vi "Test DAQ Synchronize.vi"() -> ()   [LabVIEW 2019, in "Instrument.Lockin.lvlib" / "Instrument.DAQ.lvclass"]
uses:
  Instrument.DAQ.lvclass
  Typedefs/DAQ.Config.AI--Cluster.ctl
  Typedefs/DAQ.Config.AI.Coupling--enum.ctl
  Typedefs/DAQ.Config.AI.Range--enum.ctl
  Typedefs/DAQ.Type--enum.ctl
  Typedefs/DAQ.Config.AO--Cluster.ctl
  Typedefs/DAQ.Config.AO.Range--enum.ctl
  Typedefs/DAQ.Sampling.Sample Mode--Ring.ctl
  Typedefs/DAQ.Sampling.Sampling--Cluster.ctl
  Instrument.DAQ.lvclass/Instrument.DAQ.ctl
  <vilib>/DAQmx/write.llb/DAQmx Write (Analog 1D Wfm NChan NSamp).vi
  <vilib>/DAQmx/read.llb/DAQmx Read (Analog 1D Wfm NChan NSamp).vi
  <vilib>/DAQmx/miscellaneous.llb/DAQmx Fill In Error Info.vi
  <vilib>/measure/NI_MABase.lvlib
  <resource>/objmgr/daqmx.rc
panel:
  out "Waveform Graph":dbl[][](graph)
  in  "stop":bool
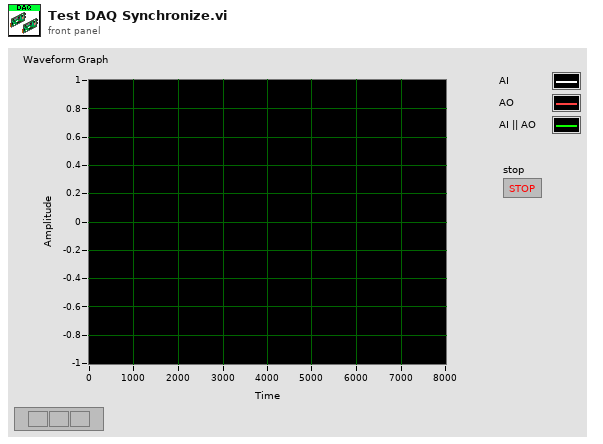
[diagram p1: front panel]
types:
  T1 = typedef "Instrument.Lockin.lvlib/Instrument.DAQ.lvclass/DAQ.Sampling.Sampling--Cluster.ctl" = cluster{"Fs":dbl, "#s":i32}
  T2 = typedef "Instrument.Lockin.lvlib/Instrument.DAQ.lvclass/DAQ.Sampling.Sample Mode--Ring.ctl" = i32
  T3 = typedef "Instrument.Lockin.lvlib/Instrument.DAQ.lvclass/DAQ.Config.AO--Cluster.ctl" = cluster{"Channels":tag, "Range":T4, "output terminal configuration":i32, "Type":T5}
  T4 = typedef "Instrument.Lockin.lvlib/Instrument.DAQ.lvclass/DAQ.Config.AO.Range--enum.ctl" = enum16{"±0.1", "±1.0", "±10.0"}
  T5 = typedef "Instrument.Lockin.lvlib/Instrument.DAQ.lvclass/DAQ.Type--enum.ctl" = enum16{"None", "USB-4431", "PXI-446x"}
  T6 = typedef "Instrument.Lockin.lvlib/Instrument.DAQ.lvclass/DAQ.Config.AI--Cluster.ctl" = cluster{"Channels":tag, "Coupling":T7, "Range":T8, "input terminal configuration":i32, "Type":T5}
  T7 = typedef "Instrument.Lockin.lvlib/Instrument.DAQ.lvclass/DAQ.Config.AI.Coupling--enum.ctl" = u16
  T8 = typedef "Instrument.Lockin.lvlib/Instrument.DAQ.lvclass/DAQ.Config.AI.Range--enum.ctl" = enum16{"±0.316", "±1.00", "±3.16", "±10.0", "±31.6", "±42.4"}
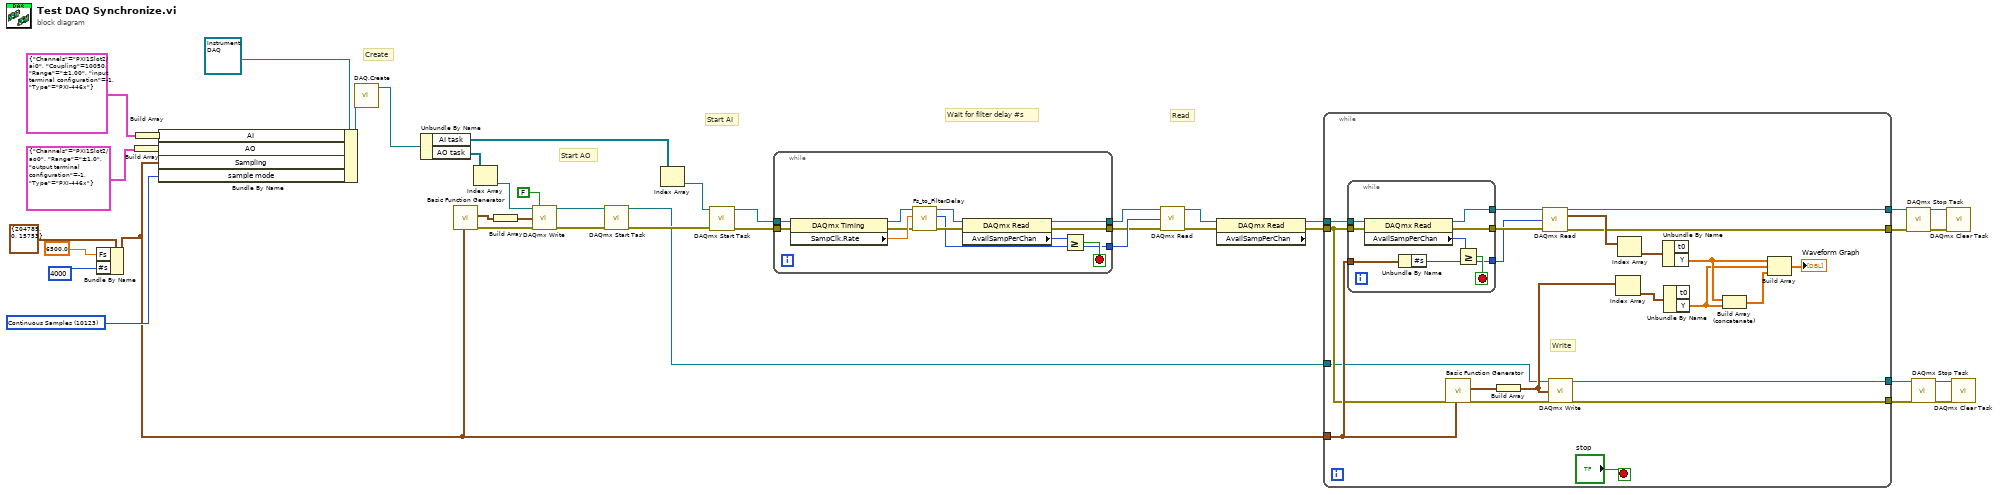
[diagram p0: block diagram]
diagram:
  w5 = T2 10123 items=["Finite Samples"=10178, "Continuous Samples"=10123] ("Configuration.DAQ.Sampling.Sample Mode")
  # "Read"
  # "Wait for filter delay #s"
  # "Start AI"
  # "Start AO"
  # "Create"
  n1 = Bundle By Name(cluster=T1 {"Fs"=204789.0, "#s"=15753} ("Configuration.DAQ.Sampling.Sampling"), "Fs"=6500.0, "#s"=4000) -> (w1:T1)
  n2 = Build Array(T3 {"Channels"="PXI1Slot2/ao0", "Range"=enum."±1.0", "output terminal configuration"=-1, "Type"=enum."PXI-446x"} ("AO.config")) -> (w16:T3[])
  n3 = Build Array(T6 {"Channels"="PXI1Slot2/ai0", "Coupling"=10050, "Range"=enum."±1.00", "input terminal configuration"=-1, "Type"=enum."PXI-446x"} ("AI.Config")) -> (w17:T6[])
  n4 = Bundle By Name(cluster=refnum<class "Instrument.DAQ.lvclass"> refnum ("Instrument.DAQ"), "AI"=w17, "AO"=w16, "Sampling"=w1, "sample mode"=w5) -> (w34:refnum<class "Instrument.DAQ.lvclass">)
  n5 = call "DAQ.Create.vi"("Instrument.DAQ"=w34) -> ("Instrument.DAQ"=w41:refnum<class "Instrument.DAQ.lvclass">)  [unwired: 9 in, 1 out]
  n6 = Unbundle By Name(w41) -> ("AI task"=w29:refnum<k21>[], "AO task"=w39:refnum<k21>[])
  n7 = call <vilib>:"Basic Function Generator.vi"("sampling info"=w1) -> ("error out"=w31:errorcluster, "signal out"=w37:waveform(dbl))  [unwired: 8 in, 1 out]
  n8 = Index Array(array=w39) -> (element=w38:refnum<k21>)  [unwired: 1 in]
  n9 = Build Array(w37) -> (w36:waveform(dbl)[])
  n10 = call-poly <vilib>:"DAQmx Write.vi"("task/channels in"=w38, "auto start"=FALSE, "data"=w36, "error in"=w31) -> ("task out"=w33:refnum<k21>, "error out"=w32:errorcluster)  [unwired: 9 in, 1 out]
  n11 = call <vilib>:"DAQmx Start Task.vi"("task/channels in"=w33, "error in"=w32) -> ("task out"=w14:refnum<k21>, "error out"=w23:errorcluster)  [unwired: 12 in]
  n12 = Index Array(array=w29) -> (element=w30:refnum<k21>)  [unwired: 1 in]
  n13 = call <vilib>:"DAQmx Start Task.vi"("task/channels in"=w30, "error in"=w23) -> ("task out"=w27:refnum<k21>, "error out"=w28:errorcluster)  [unwired: 12 in]
  n14 = while {
    tunnel: w28 -> [w46]
    tunnel: w27 -> [w47]
    tunnel: [w51] -> w24
    tunnel: [w42] -> w26
    tunnel: [w50] -> w25
    stop <- w52 stop-if-true
    n15 = property class="DAQmx Timing"(reference=w47, error in=w46) -> (reference out=w45:refnum<k21>, error out=w48:errorcluster, "SampClk.Rate"=w49:dbl)
    n16 = call "Fs_to_FilterDelay.vi"("error in (no error)"=w48, "Fs"=w49, "Refnum in"=w45) -> ("error out"=w43:errorcluster, "Total Filter Delay (samples)"=w42:i32, "Refnum out"=w44:refnum<k21>)  [unwired: 6 in]
    n17 = property class="DAQmx Read"(reference=w44, error in=w43) -> (reference out=w51:refnum<k21>, error out=w50:errorcluster, "AvailSampPerChan"=w53:u32)
    n18 = Greater Or Equal?(x=w53, y=w42) -> (x >= y?=w52:bool)
  }
  n19 = call-poly <vilib>:"DAQmx Read.vi"("task/channels in"=w24, "number of samples per channel"=w26, "error in"=w25) -> ("task out"=w22:refnum<k21>, "error out"=w21:errorcluster)  [unwired: 10 in, 1 out]
  n20 = property class="DAQmx Read" props=["AvailSampPerChan"](reference=w22, error in=w21) -> (reference out=w20:refnum<k21>, error out=w19:errorcluster)  [unwired: 1 out]
  n21 = while {
    tunnel: w20 -> [w75]
    tunnel: w19 -> [w70]
    tunnel: w14 -> [w59]
    tunnel: w1 -> [w71]
    tunnel: [w58] -> w13
    tunnel: [w57] -> w12
    tunnel: [w56] -> w7
    tunnel: [w55] -> w6
    stop <- "stop" stop-if-true
    # "Write"
    n22 = while {
      tunnel: w75 -> [w83]
      tunnel: w70 -> [w82]
      tunnel: [w81] -> w74
      tunnel: [w80] -> w73
      tunnel: w71 -> [w77]
      tunnel: [w76] -> w54
      stop <- w78 stop-if-true
      n23 = property class="DAQmx Read"(reference=w83, error in=w82) -> (reference out=w81:refnum<k21>, error out=w80:errorcluster, "AvailSampPerChan"=w79:u32)
      n24 = Unbundle By Name(w77) -> ("#s"=w76:i32)
      n25 = Greater Or Equal?(x=w79, y=w76) -> (x >= y?=w78:bool)
    }
    n26 = call <vilib>:"Basic Function Generator.vi"("sampling info"=w71, "error in (no error)"=w70) -> ("error out"=w60:errorcluster, "signal out"=w72:waveform(dbl))  [unwired: 7 in, 1 out]
    n27 = Build Array(w72) -> (w63:waveform(dbl)[])
    n28 = call-poly <vilib>:"DAQmx Read.vi"("task/channels in"=w74, "number of samples per channel"=w54, "error in"=w73) -> ("task out"=w58:refnum<k21>, "data"=w64:waveform(dbl)[], "error out"=w57:errorcluster)  [unwired: 10 in]
    n29 = call-poly <vilib>:"DAQmx Write.vi"("task/channels in"=w59, "data"=w63, "error in"=w60) -> ("task out"=w56:refnum<k21>, "error out"=w55:errorcluster)  [unwired: 10 in, 1 out]
    n30 = Index Array(array=w63) -> (element=w66:waveform(dbl))  [unwired: 1 in]
    n31 = Index Array(array=w64) -> (element=w65:waveform(dbl))  [unwired: 1 in]
    n32 = Unbundle By Name(w65) -> ("Y"=w62:dbl[])  [unwired: 1 out]
    n33 = Unbundle By Name(w66) -> ("Y"=w61:dbl[])  [unwired: 1 out]
    n34 = Build Array (concatenate)(w62, w61) -> (w68:dbl[])
    n35 = Build Array(w62, w61, w68) -> (→"Waveform Graph":dbl[][])
  }
  n36 = call <vilib>:"DAQmx Stop Task.vi"("task/channels in"=w13, "error in"=w12) -> ("task out"=w10:refnum<k21>, "error out"=w11:errorcluster)  [unwired: 12 in]
  n37 = call <vilib>:"DAQmx Stop Task.vi"("task/channels in"=w7, "error in"=w6) -> ("task out"=w9:refnum<k21>, "error out"=w8:errorcluster)  [unwired: 12 in]
  n38 = call <vilib>:"DAQmx Clear Task.vi"("task in"=w10, "error in"=w11) -> ()  [unwired: 13 in, 1 out]
  n39 = call <vilib>:"DAQmx Clear Task.vi"("task in"=w9, "error in"=w8) -> ()  [unwired: 13 in, 1 out]
